vi "AG34980A_DAC_Apply_Level.vi"(0 "VISA resource name":refnum<visa-resource-name>, 1 "Channel List":string, 5 "Source Type (0:Voltage)":enum16{"Voltage", "Current"}(ring), 9 "Level":dbl, 11 "error in (no error)":errorcluster, 12 "Module Type (0:34952A)":enum16{"34952A", "34951A"}(ring)) -> (4 "VISA resource name out":refnum<visa-resource-name>, 15 "error out":errorcluster)   [LabVIEW 2019]
doc: "This VI allows you to apply a level voltage or current to one or more channels on the 34951A Isolated DAC module."
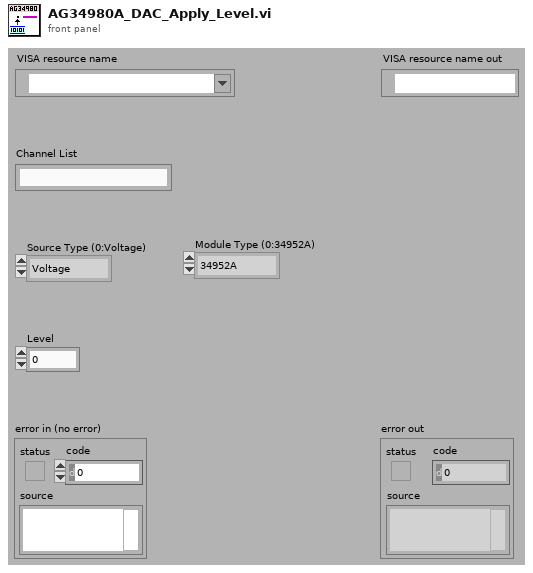
[diagram p1: front panel]
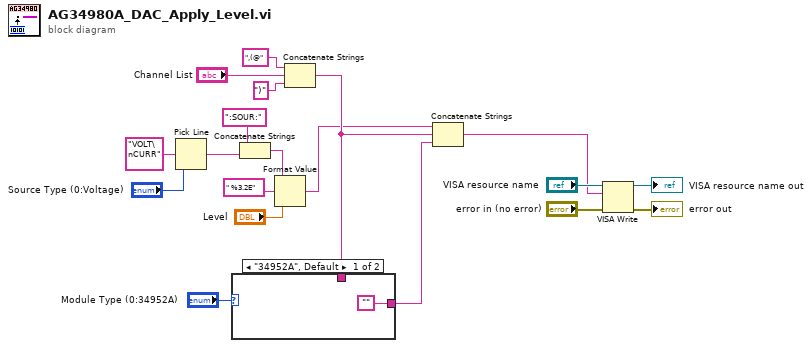
[diagram p0: block diagram]
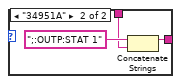
[diagram p2: hidden frame]
diagram:
  n1 = Pick Line(multi-line string="VOLT\nCURR", line index="Source Type (0:Voltage)") -> (output string=w6:string)  [unwired: 1 in]
  n2 = Concatenate Strings(":SOUR:", w6) -> (w5:string)
  n3 = Format Value(string ("")=w5, format string=" %3.2E", value (0)="Level") -> (output string=w3:string)
  n4 = Concatenate Strings(",(@", "Channel List", ")") -> (w19:string)
  n5 = case shown="\"34952A\", Default" "Module Type (0:34952A)" {
    tunnel: ["" w21] -> w2
    tunnel: w19 -> [_ w22]
    frame "34952A", Default {
    }
    frame "34951A" {
      n6 = Concatenate Strings(";:OUTP:STAT 1", w22) -> (w21:string)
    }
  }
  n7 = Concatenate Strings(w3, w19, w2) -> (w11:string)
  n8 = VISA Write(VISA resource name="VISA resource name", write buffer=w11, error in (no error)="error in (no error)") -> (VISA resource name out=→"VISA resource name out":refnum<visa-resource-name>, error out=→"error out":errorcluster)  [unwired: 1 out]
